vi "update_parameters.vi"(1 "learning_rate":dbl, 2 "grads":map{string, dbl[][]}(c390), 3 "parameters":map{string, dbl[][]}(c390)) -> (0 "train_params":map{string, dbl[][]}(c390))   [LabVIEW 2020]
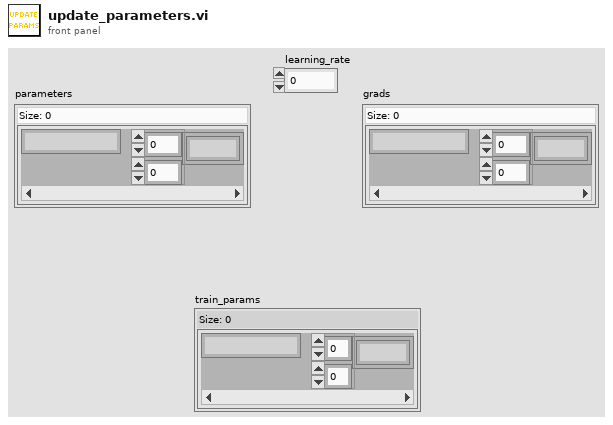
[diagram p1: front panel]
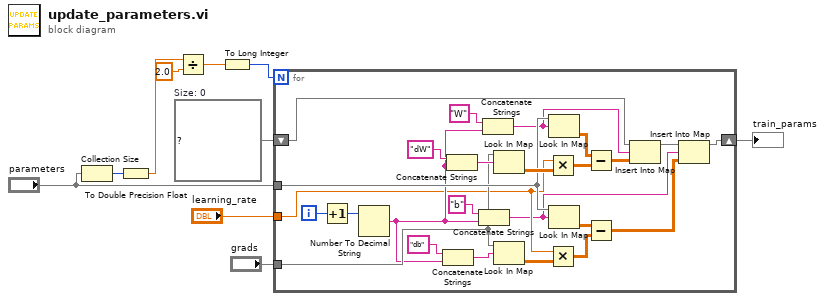
[diagram p0: block diagram]
diagram:
  w2 = map{string, dbl[][]} {}  # Size: 0
  n1 = Collection Size(1:"parameters") -> (0:w10:i32)
  n2 = To Double Precision Float(number=w10) -> (double precision float=w9:dbl)
  n3 = Divide(x=w9, y=2.0) -> (x/y=w7:dbl)
  n4 = To Long Integer(number=w7) -> (32bit integer=w6:i32)
  n5 = for {
    N: w6 -> [_]
    tunnel: "parameters" -> [w26]
    tunnel: "grads" -> [w23]
    tunnel: "learning_rate" -> [w19]
    shift-right: [w11] -> w1
    shift-left: w2 -> [w17]
    i -> [w35]
    n6 = Increment(x=w35) -> (x+1=w34:i32)
    n7 = Number To Decimal String(number=w34) -> (decimal integer string=w21:string)  [unwired: 1 in]
    n8 = Concatenate Strings("db" ("string"), w21) -> (w22:string)
    n9 = Concatenate Strings("dW" ("string"), w21) -> (w31:string)
    n10 = Concatenate Strings("b" ("string"), w21) -> (w12:string)
    n11 = Concatenate Strings("W" ("string"), w21) -> (w16:string)
    n12 = Look In Map(map=w23, key=w31) -> (value=w29:dbl[][])  [unwired: 1 in, 1 out]
    n13 = Look In Map(map=w23, key=w22) -> (value=w18:dbl[][])  [unwired: 1 in, 1 out]
    n14 = Multiply(x=w19, y=w29) -> (x*y=w28:dbl[][])
    n15 = Multiply(x=w19, y=w18) -> (x*y=w24:dbl[][])
    n16 = Look In Map(map=w26, key=w16) -> (value=w32:dbl[][])  [unwired: 1 in, 1 out]
    n17 = Look In Map(map=w26, key=w12) -> (value=w25:dbl[][])  [unwired: 1 in, 1 out]
    n18 = Subtract(x=w32, y=w28) -> (x-y=w15:dbl[][])
    n19 = Subtract(x=w25, y=w24) -> (x-y=w13:dbl[][])
    n20 = Insert Into Map(map in=w17, key=w16, value=w15) -> (map out=w14:map{string, dbl[][]})  [unwired: 2 out]
    n21 = Insert Into Map(map in=w14, key=w12, value=w13) -> (map out=w11:map{string, dbl[][]})  [unwired: 2 out]
  }
  "train_params" <- w1
